vi "Camera New Frame Arrived Callback.vi"(4 "Camera_Prime95B in":refnum<class "Camera_Prime95B.lvclass">, 5 "Event Data":cluster{"sender":refnum<k24>, "e":refnum<k24>}, 6 "Control Ref":refnum<k24>, 7 "Event Common Data":T1) -> ()   [LabVIEW 2020, in "Camera_Prime95B.lvlib" / "Camera_Prime95B.lvclass"]
uses:
  Camera_Prime95B.lvclass
  E:/Development/DevHardSoftware/MMicroscopyAF/Model/Real Hardware/Camera_Prime95B/Camera_Prime95B/Dependencies/PVCamNET.dll
  Dependencies/PVCamNET.dll
  Camera_Prime95B.lvclass/Camera_Prime95B.ctl
  Camera Prime95B Controller Messages/Update UI Msg/Update UI Msg.lvclass/Update UI Msg.ctl
  <vilib>/ActorFramework/Message Enqueuer/Message Enqueuer.lvclass/Message Enqueuer.ctl
  <vilib>/ActorFramework/Message Enqueuer/Enqueue.vi
  Camera Prime95B Controller Messages/Update UI Msg/Update UI Msg.lvclass
  C:/Program Files/National Instruments/LabVIEW 2020/vi.lib/ActorFramework/Message/Message.lvclass
  <vilib>/ActorFramework/Message Priority Queue/Priority Enqueue.vi
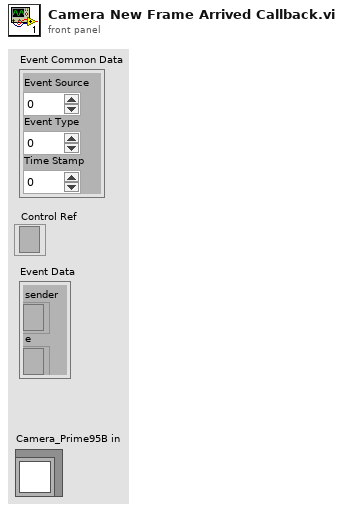
[diagram p1: front panel]
types:
  T1 = cluster{"Event Source":i32, "Event Type":u32, "Time Stamp":u32}
  T2 = typedef "Image Type" = u32
  T3 = typedef "IMAQ Image.ctl" = refnum<image>
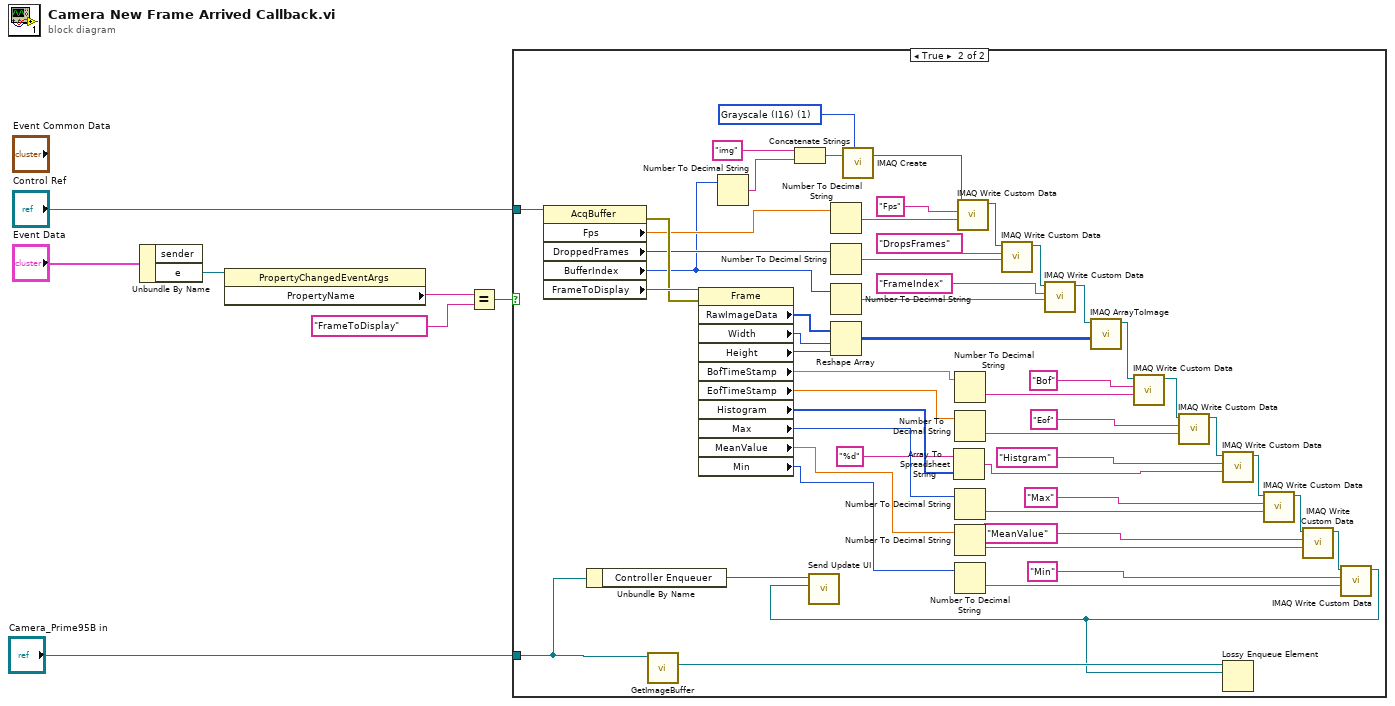
[diagram p0: block diagram]
diagram:
  n1 = Unbundle By Name("Event Data") -> ("e"=w6:refnum<k24>)  [unwired: 1 out]
  n2 = property class="PropertyChangedEventArgs"(reference=w6) -> ("PropertyName"=w5:string)  [unwired: 1 in, 2 out]
  n3 = Equal?(x=w5, y="FrameToDisplay") -> (x = y?=w3:bool)
  n4 = case shown="True" w3 {
    tunnel: "Control Ref" -> [_ w60]
    tunnel: "Camera_Prime95B in" -> [_ w10]
    frame False {
    }
    frame True {
      w54 = T2 1 items=["Grayscale (U8)", "Grayscale (I16)", "Grayscale (SGL)", "Complex (CSG)", "RGB (U32)", "HSL (U32)", "RGB (U64)", "Grayscale (U16)"] ("Image Type")
      n5 = property class="AcqBuffer"(reference=w60) -> (error out=w58:errorcluster, "Fps"=w24:sgl, "DroppedFrames"=w23:i32, "BufferIndex"=w15:i32, "FrameToDisplay"=w59:refnum<k24>)  [unwired: 1 in, 1 out]
      n6 = Unbundle By Name(w10) -> ("Controller Enqueuer"=w9:refnum<class "Message Enqueuer.lvclass">)
      n7 = call-dynamic "GetImageBuffer.vi"("Camera in"=w10) -> ("ImageBuffers"=w11:refnum<queue>)  [unwired: 8 in, 2 out]
      n8 = property class="Frame"(reference=w59, error in=w58) -> ("RawImageData"=w53:i16[], "Width"=w52:u32, "Height"=w51:u32, "BofTimeStamp"=w49:dbl, "EofTimeStamp"=w31:dbl, "Histogram"=w29:u32[], "Max"=w30:u32, "MeanValue"=w26:dbl, "Min"=w25:u32)  [unwired: 2 out]
      n9 = Number To Decimal String(number=w15) -> (decimal integer string=w57:string)  [unwired: 1 in]
      n10 = Concatenate Strings("img" ("Image Name"), w57) -> (w55:string)
      n11 = Number To Decimal String(number=w24) -> (decimal integer string=w20:string)  [unwired: 1 in]
      n12 = Number To Decimal String(number=w23) -> (decimal integer string=w17:string)  [unwired: 1 in]
      n13 = Number To Decimal String(number=w15) -> (decimal integer string=w16:string)  [unwired: 1 in]
      n14 = Reshape Array(w53, w52, w51) -> (w50:i16[][])
      n15 = call "IMAQ Create"("Image Name"=w55, "Image Type"=w54) -> ("New Image"=w22:T3)  [unwired: 3 in, 1 out]
      n16 = Array To Spreadsheet String(array=w29, 3:"%d" ("format string")) -> (spreadsheet string=w27:string)  [unwired: 1 in]
      n17 = Number To Decimal String(number=w49) -> (decimal integer string=w48:string)  [unwired: 1 in]
      n18 = Number To Decimal String(number=w31) -> (decimal integer string=w46:string)  [unwired: 1 in]
      n19 = Number To Decimal String(number=w30) -> (decimal integer string=w43:string)  [unwired: 1 in]
      n20 = Number To Decimal String(number=w26) -> (decimal integer string=w41:string)  [unwired: 1 in]
      n21 = Number To Decimal String(number=w25) -> (decimal integer string=w39:string)  [unwired: 1 in]
      n22 = call "IMAQ Write Custom Data"("Custom Data In"=w20, "Key"="Fps", "Image"=w22) -> ("Image Out"=w18:T3)  [unwired: 7 in, 1 out]
      n23 = call "IMAQ Write Custom Data"("Custom Data In"=w17, "Key"="DropsFrames", "Image"=w18) -> ("Image Out"=w12:T3)  [unwired: 7 in, 1 out]
      n24 = call "IMAQ Write Custom Data"("Custom Data In"=w16, "Key"="FrameIndex", "Image"=w12) -> ("Image Out"=w13:T3)  [unwired: 7 in, 1 out]
      n25 = call "IMAQ ArrayToImage"("Image Pixels (I16)"=w50, "Image"=w13) -> ("Image Out"=w37:T3)  [unwired: 8 in, 1 out]
      n26 = call "IMAQ Write Custom Data"("Custom Data In"=w48, "Key"="Bof", "Image"=w37) -> ("Image Out"=w36:T3)  [unwired: 7 in, 1 out]
      n27 = call "IMAQ Write Custom Data"("Custom Data In"=w46, "Key"="Eof", "Image"=w36) -> ("Image Out"=w35:T3)  [unwired: 7 in, 1 out]
      n28 = call "IMAQ Write Custom Data"("Custom Data In"=w27, "Key"="Histgram", "Image"=w35) -> ("Image Out"=w34:T3)  [unwired: 7 in, 1 out]
      n29 = call "IMAQ Write Custom Data"("Custom Data In"=w43, "Key"="Max", "Image"=w34) -> ("Image Out"=w33:T3)  [unwired: 7 in, 1 out]
      n30 = call "IMAQ Write Custom Data"("Custom Data In"=w41, "Key"="MeanValue", "Image"=w33) -> ("Image Out"=w32:T3)  [unwired: 7 in, 1 out]
      n31 = call "IMAQ Write Custom Data"("Custom Data In"=w39, "Key"="Min", "Image"=w32) -> ("Image Out"=w8:T3)  [unwired: 7 in, 1 out]
      n32 = call "Send Update UI.vi"("Image In"=w8, "Message Enqueuer"=w9) -> ()  [unwired: 8 in, 2 out]
      n33 = Lossy Enqueue Element(queue=w11, element=w8) -> ()  [unwired: 1 in, 4 out]
    }
  }
